vi "GUI_StagingAlignCam.vi"() -> ()   [LabVIEW 2013]
uses:
  shared programs/GUI_Template/GUI_master/tcp_new_data_event.ctl
  shared programs/GUI_Template/GUI_master/tcp new data cluster.ctl
  <vilib>/vision/Image Controls.llb/IMAQ Image.ctl
  <vilib>/vision/NI_Vision_Development_Module.lvlib
panel:
  in  "abort::2":bool
  in  "xpos::2":dbl
  in  "GUIdevice 2":string="StagingHexapodPI"
  out "error out":errorcluster
  out "image2":T1(plugin-control) caption="StagingM1Near"
  in  "Parameters":T2={"Operator"=enum."Square", "X Value"=1.5} {"X Value" format="%.2f"}
  out "tcp data event":T3
  out "error IO 2":errorcluster
  out "image::1":T1(plugin-control) caption="StagingModeTemp"
  in  "GUIdevice 1":string="TS-StagingAlignment"
  in  "insert tag":bool=TRUE
  in  "stop":bool
  # "(for Power X and \nPower 1/X only)"
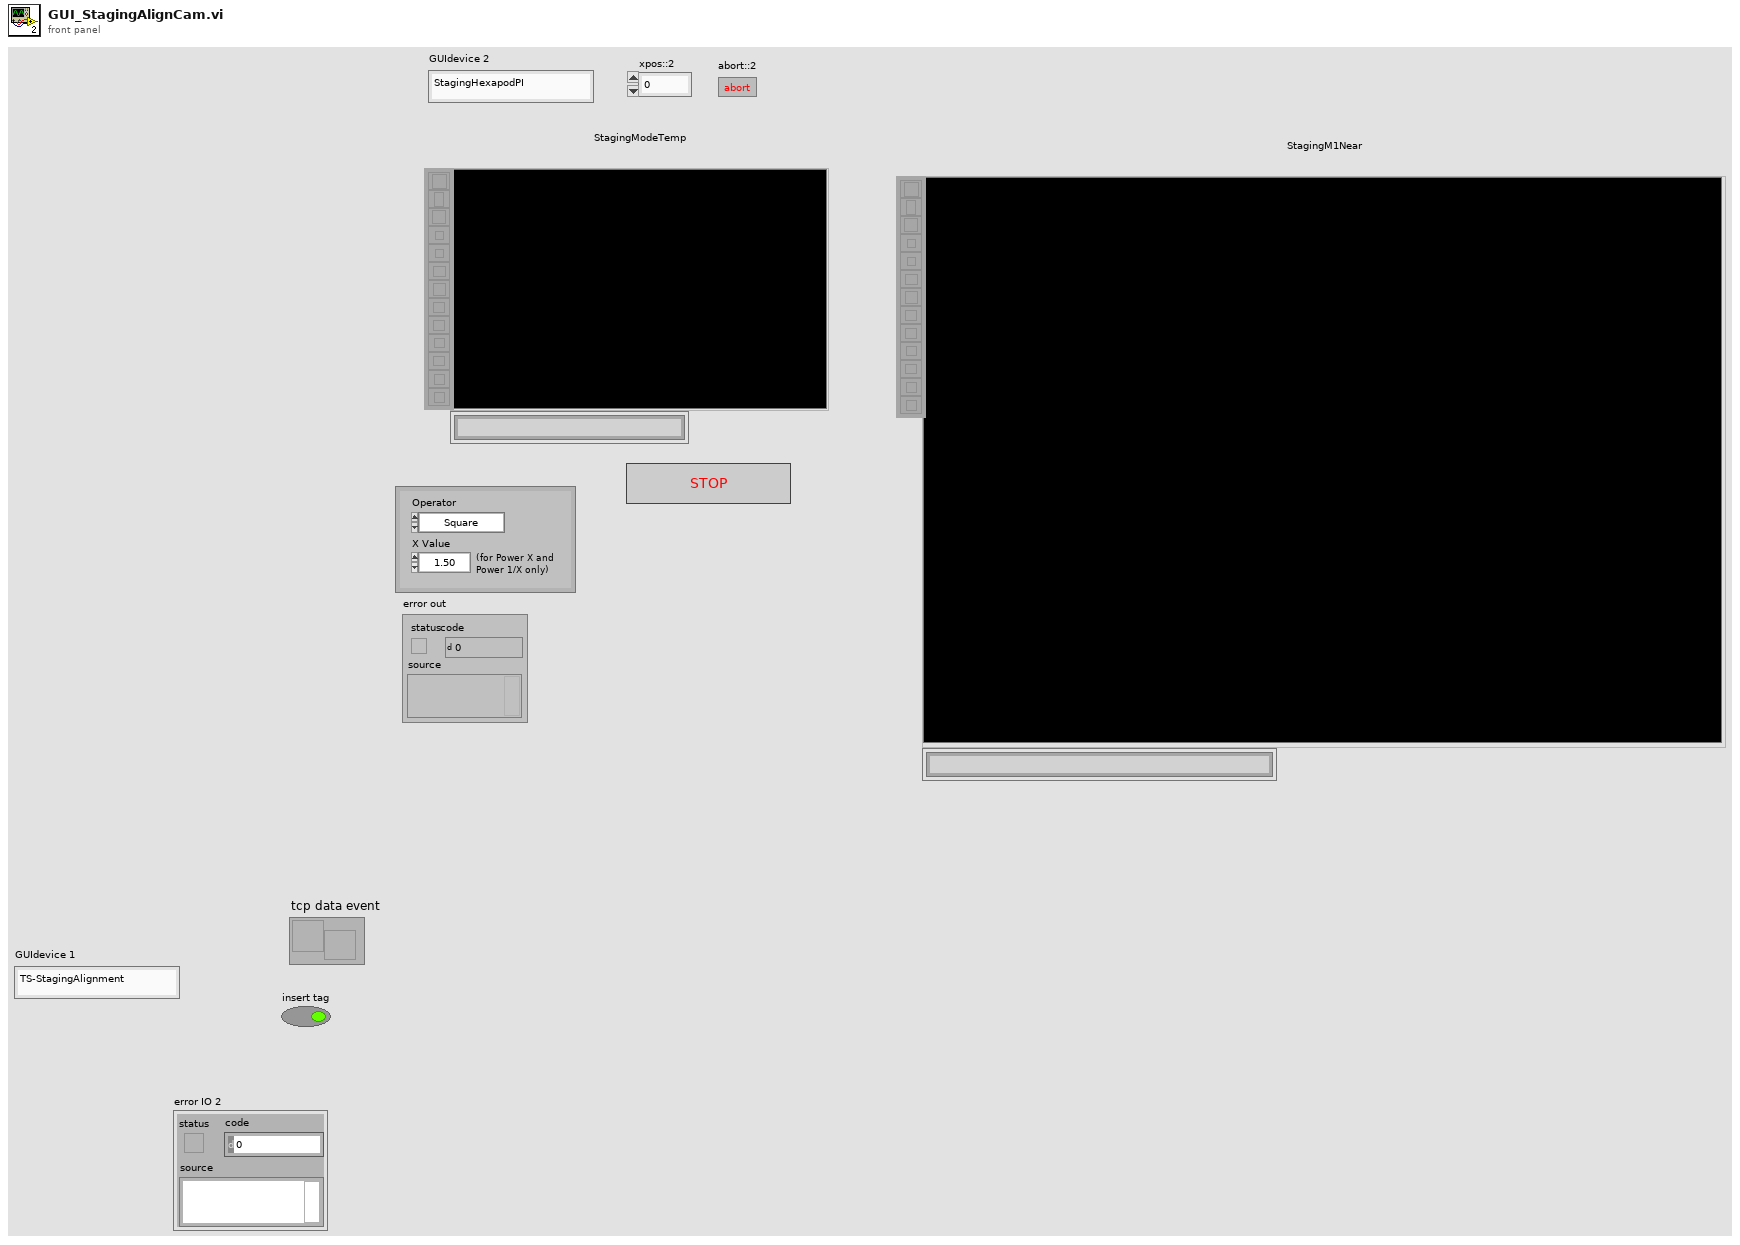
[diagram p1: front panel]
types:
  T1 = typedef "IMAQ Image.ctl" = refnum<image>
  T2 = cluster{"Operator":enum32{"Linear", "Log", "Exp", "Square", "Square root", "Power X", "Power 1/X"}, "X Value":sgl}
  T3 = typedef "tcp_new_data_event.ctl" = refnum<user-event>
  T4 = typedef "Image Type" = u32
  T5 = typedef "tcp new data cluster.ctl" = cluster{"EventEnum":enum16{"new data", "connection status update"}, "Device name":string}
  T6 = enum32{"Linear", "Log", "Exp", "Square", "Square root", "Power X", "Power 1/X"}
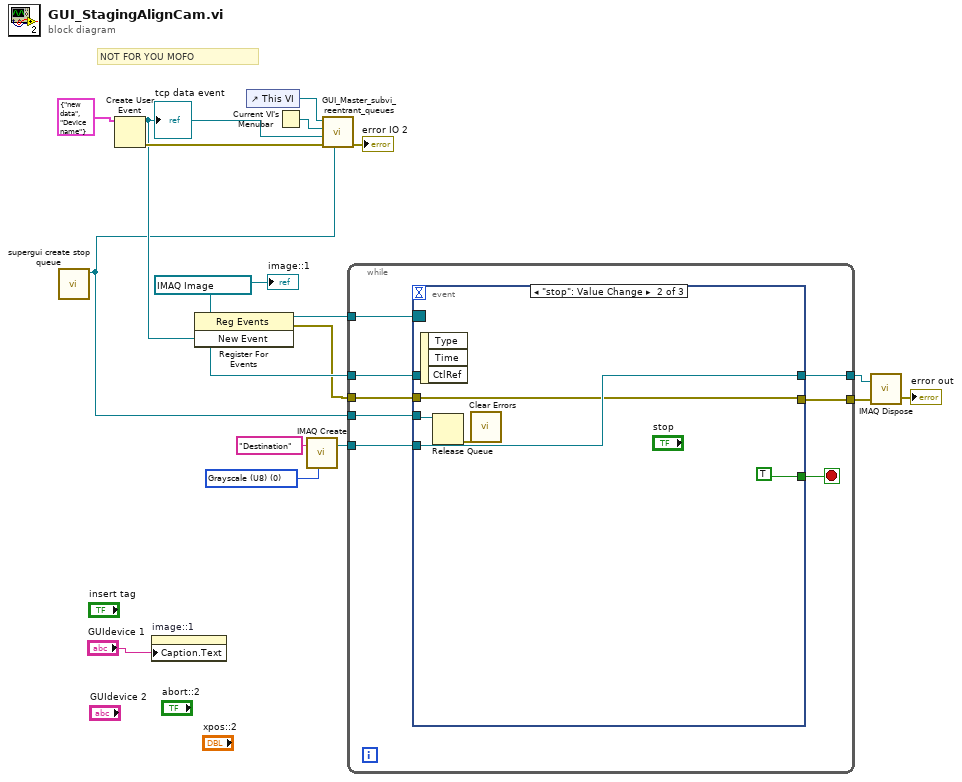
[diagram p0: block diagram]
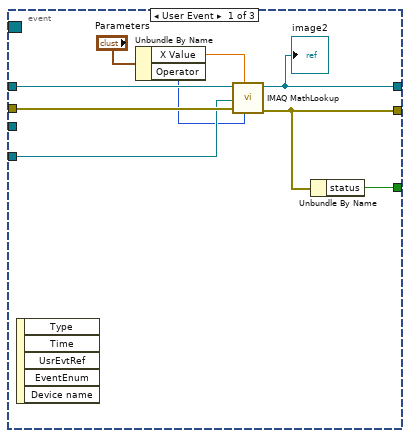
[diagram p2: hidden frame]
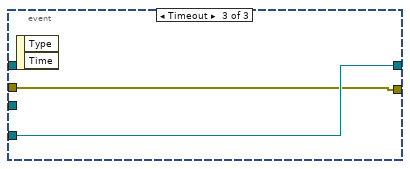
[diagram p3: hidden frame]
diagram:
  w2 = T4 0 items=["Grayscale (U8)", "Grayscale (I16)", "Grayscale (SGL)", "Complex (CSG)", "RGB (U32)", "HSL (U32)", "RGB (U64)", "Grayscale (U16)"] ("Image Type")
  w9 = T1 refnum ("New Image")
  # "NOT FOR YOU MOFO"
  n1 = call "supergui create stop queue.vi"() -> ("STOP Queue out"=w1:refnum<queue>)  [unwired: 11 in]
  n2 = Create User Event(user event datatype=T5 {"EventEnum"=enum."new data", "Device name"="Device name"} ("New Event")) -> (user event=w5:refnum<user-event>, error out=w13:errorcluster)  [unwired: 1 in]
  "tcp data event" <- w5
  n3 = property on="image::1" class="ImageControl"("Caption.Text"="GUIdevice 1") -> ()  [unwired: 2 in, 2 out]
  n4 = register-events(w5) -> (reference out=w6:refnum<event-registration>, error out=w4:errorcluster)  [unwired: 2 in]
  n5 = control-ref of="This VI"() -> (w16:refnum<vi>)
  n6 = Current VI's Menubar() -> (w15:refnum<k9>)
  n7 = call "IMAQ Create"("Image Name"="Destination", "Image Type"=w2) -> ("New Image"=w10:T1)  [unwired: 2 in, 2 out]
  n8 = call "GUI_Master_subvi_reentrant_queues.vi"("STOP Queue in"=w1, "error in (no error)"=w13, "tcp data event"=w5, "Caller menu reference"=w15, "Caller VI ref"=w16) -> ("error out"=→"error IO 2":errorcluster)  [unwired: 6 in]
  n9 = while {
    tunnel: w9 -> [w23]
    tunnel: w4 -> [w25]
    tunnel: w10 -> [w24]
    tunnel: [w21] -> w8
    tunnel: [w22] -> w7
    tunnel: w6 -> [w19]
    tunnel: w1 -> [w18]
    stop <- w20 stop-if-true
    n10 = event shown="[1] \"stop\": Value Change" {
      selector: w19 -> [_ _ _]
      dyn-events: _ -> [_ _ _]
      timeout: _ -> [_ _ _]
      tunnel: w25 -> [w33 w37 w40]
      tunnel: w24 -> [w32 w38 w41]
      tunnel: w23 -> [w31 _ _]
      tunnel: [w27 w37 w40] -> w22
      tunnel: [w30 w38 w41] -> w21
      tunnel: [w26 TRUE ("stop") _] -> w20
      tunnel: w18 -> [_ w36 _]
      event User Event {
        n11 = event-data() -> ()  [unwired: 1 in, 5 out]
        n12 = Unbundle By Name("Parameters") -> ("X Value"=w28:sgl, "Operator"=w29:T6)
        n13 = call "IMAQ MathLookup"("Operator"=w29, "X Value"=w28, "error in (no error)"=w33, "Image Dst"=w32, "Image Src"=w31) -> ("error out"=w27:errorcluster, "Image Dst Out"=w30:T1)  [unwired: 2 in, 3 out]
        "image2" <- w30
        n14 = Unbundle By Name(w27) -> ("status"=w26:bool)
      }
      event "stop": Value Change {
        n15 = event-data() -> ()  [unwired: 1 in, 3 out]
        n16 = Release Queue(queue=w36) -> (error out=w35:errorcluster)  [unwired: 2 in, 2 out]
        n17 = call <vilib>:"Clear Errors.vi"("error in (no error)"=w35) -> ()  [unwired: 6 in, 1 out]
      }
      event Timeout {
        n18 = event-data() -> ()  [unwired: 1 in, 2 out]
      }
    }
  }
  n19 = call "IMAQ Dispose"("Image"=w8, "error in (no error)"=w7) -> ("error out"=→"error out":errorcluster)  [unwired: 1 in, 3 out]
  "image::1" <- w9
